vi "Action Worker Mode Example.vi"() -> ()   [LabVIEW 2017, in "Action Worker Mode Example.lvlib"]
uses:
  Action Worker Mode Example.lvlib
  user.lib/_NEVSTOP/Communicable State Machine(CSM)/_Support/Typedef/_CSM_Response Source Message.ctl
  user.lib/_NEVSTOP/Communicable State Machine(CSM)/_Support/Typedef/_CSM_MODE.ctl
  user.lib/_NEVSTOP/Communicable State Machine(CSM)/AdvanceAPI/CSM - Make String Arguments Safe.vi
  user.lib/_NEVSTOP/Communicable State Machine(CSM)/AdvanceAPI/CSM - Break Down Multiple States String.vi
  user.lib/_NEVSTOP/Communicable State Machine(CSM)/AdvanceAPI/CSM - Compact Multiple States.vi
  user.lib/_NEVSTOP/Communicable State Machine(CSM)/AdvanceAPI/CSM - Keywords.vi
  user.lib/_NEVSTOP/Communicable State Machine(CSM)/Communicable State Machine.lvlib
panel:
  in  "All?":bool
  out "Array":T2(array[cluster])
  out ">> Response Source Message >>":T3
  in  "DoSth: Error -> Worker":bool
  in  "DoSth: Error -@ Worker":bool
  in  "Macro: Exit -> Worker":bool
  in  "Macro: Exit -@ Worker":bool
  in  "DoSth: DoA -@ Worker":bool
  out "State History":string
  in  "DoSth: DoA -> Worker":bool
  # "Overview:\n\nThis demonstrates the worker mode in the CSM framework. Worker mode involves starting multiple clonable instances of CSM, which work together as sub-modules. Normally, if we use the same name for cloneable modules, a critical error will occur in the subsequently started instance. To distinguish it from normal cases, CSM uses a # postfix in module names. Suppose the workers are named with \"worker#\". If you try to send a message to \"worker\", the first idle instance will respond to the message. The term \"FIRST IDLE\" refers to using a fairy queue for waiting instances. From outside, you won't even know that 4 worker instances are running. All concepts of CSM remain unchanged in worker mode, including sync/async/status messages.\n\nIn this example, 4 worker instances of “worker” are running in the background. Please refer to the history log to identify which instance processed your message."
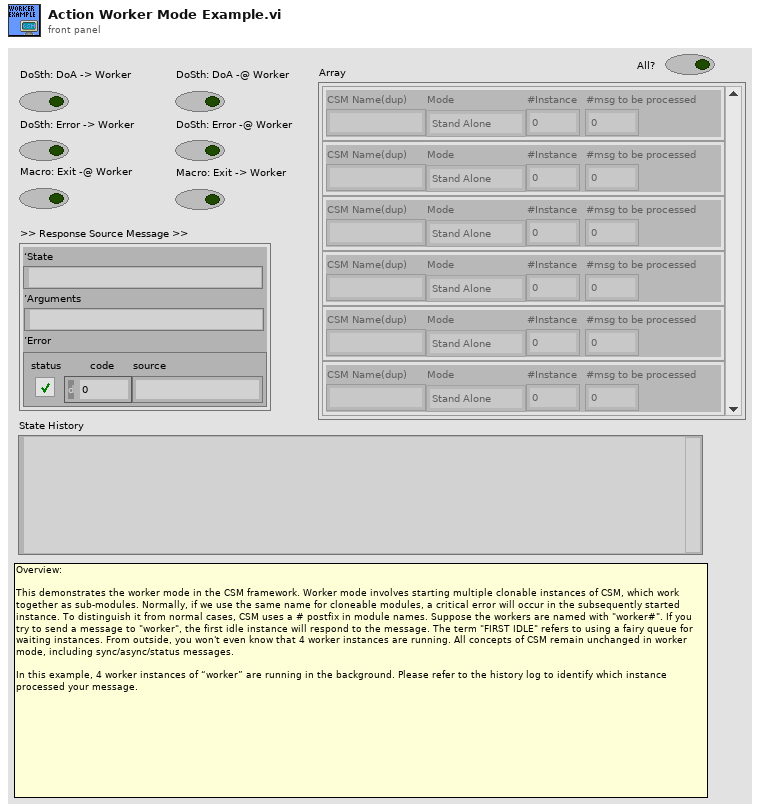
[diagram p1: front panel]
types:
  T1 = typedef "Communicable State Machine.lvlib/_CSM_MODE.ctl" = enum16{"Not Exist", "Stand Alone", "CSM", "Worker", "Worker Agent", "Chain Node", "Chain"}
  T2 = cluster{"CSM Name(dup)":string, "Mode":T1, "#Instance":i32, "#msg to be processed":i32}[]
  T3 = typedef "Communicable State Machine.lvlib/_CSM_Response Source Message.ctl" = cluster{"‘State":string, "’Arguments":string, "’Error":errorcluster}
  T4 = enum32{"Invalid", "Standard", "Closed", "Hidden", "Minimized", "Maximized"}
  T5 = enum32{"invalid app kind", "Development System", "Run Time System", "Student Edition", "Embedded LabVIEW", "Evaluation", "Custom"}
  T6 = cluster{"Current VI Reference":refnum<vi>, "Close Panel on Exit?":bool}
  T7 = cluster{"Core":cluster{"Current VI Reference":refnum<vi>, "Close Panel on Exit?":bool}, "Your Boolean data":bool, "Your string data":string}
  T8 = cluster{"CSM Name (Dup)":string, "Mode":T1, "#Instance":i32, "#Elements In Queue":i32}
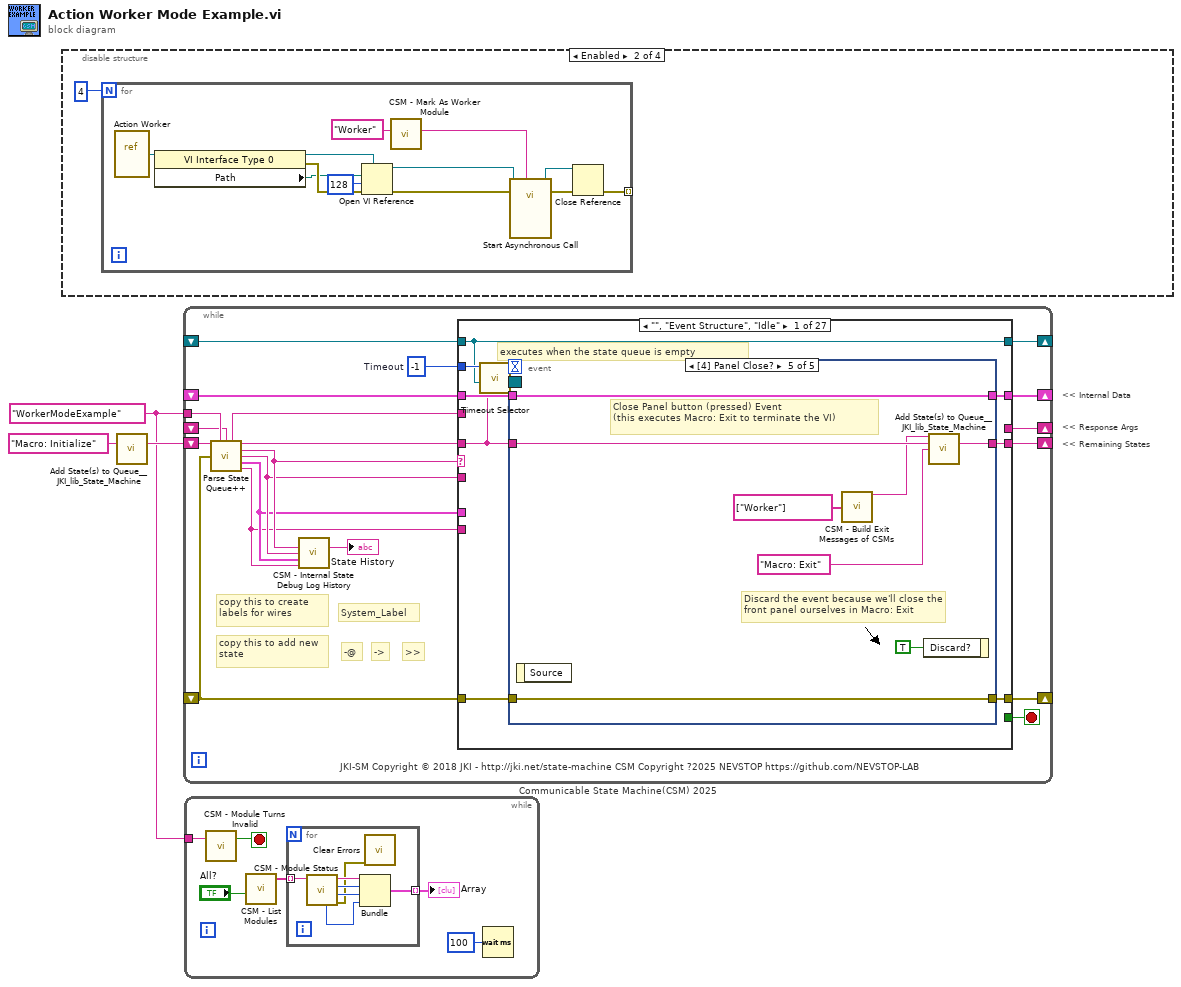
[diagram p0: block diagram]
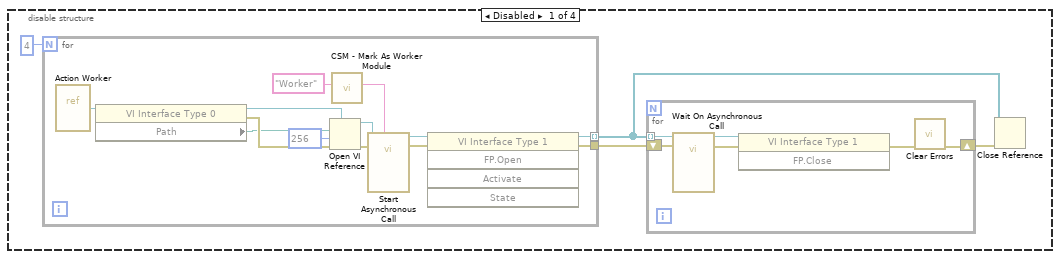
[diagram p2: hidden frame]
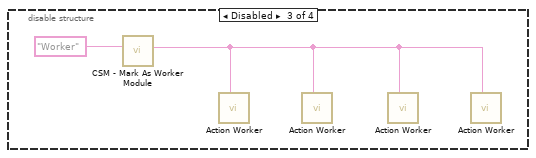
[diagram p3: hidden frame]
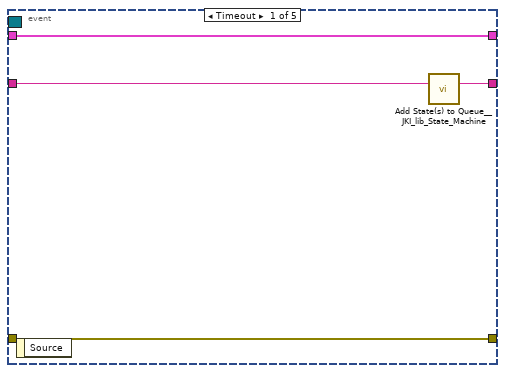
[diagram p5: hidden frame]
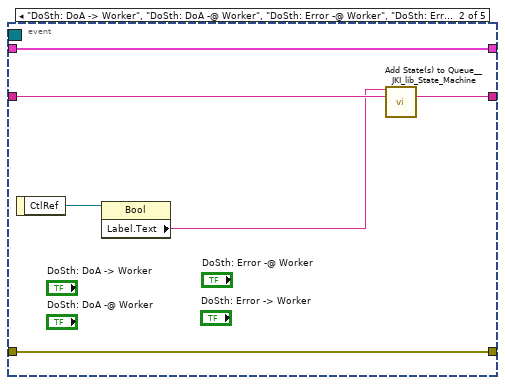
[diagram p6: hidden frame]
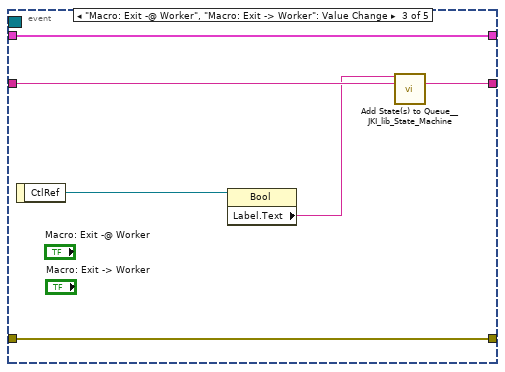
[diagram p7: hidden frame]
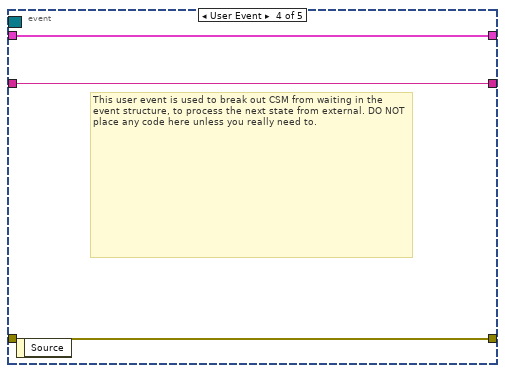
[diagram p8: hidden frame]
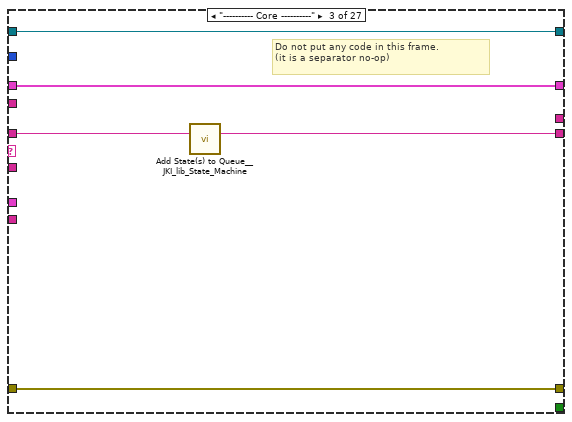
[diagram p10: hidden frame]
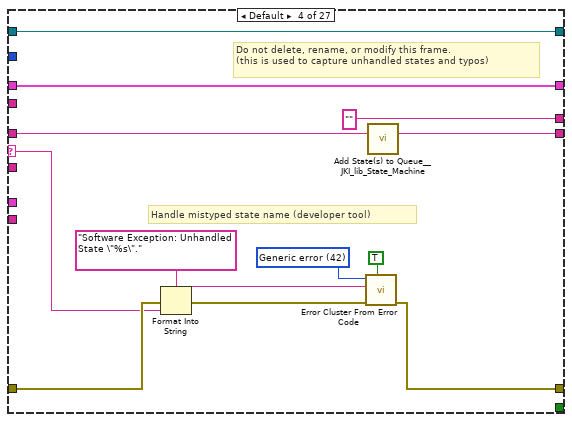
[diagram p11: hidden frame]
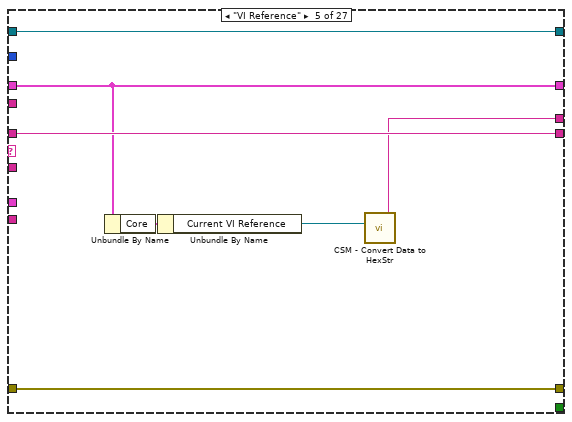
[diagram p12: hidden frame]
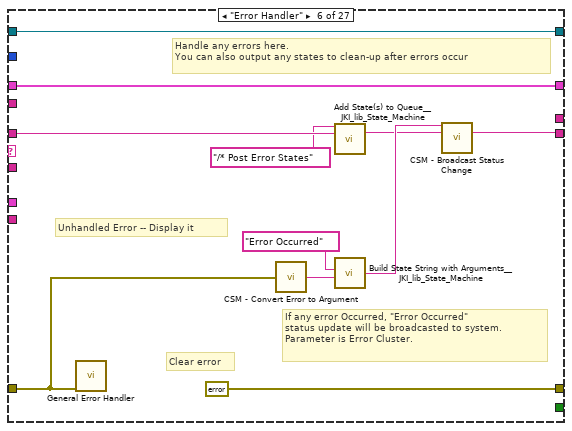
[diagram p13: hidden frame]
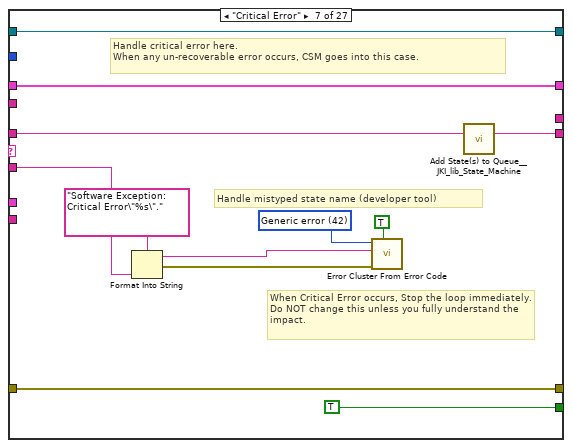
[diagram p14: hidden frame]
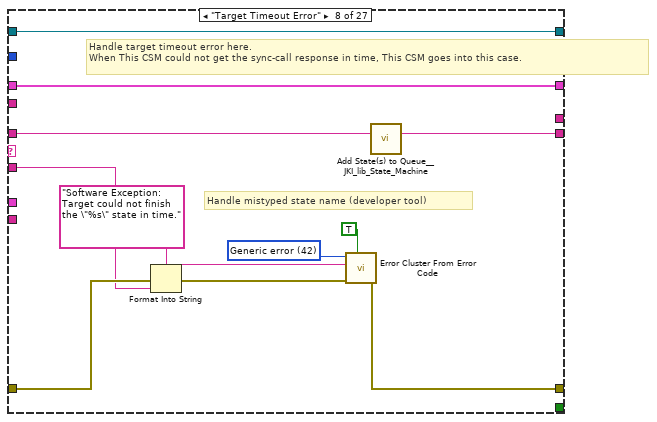
[diagram p15: hidden frame]
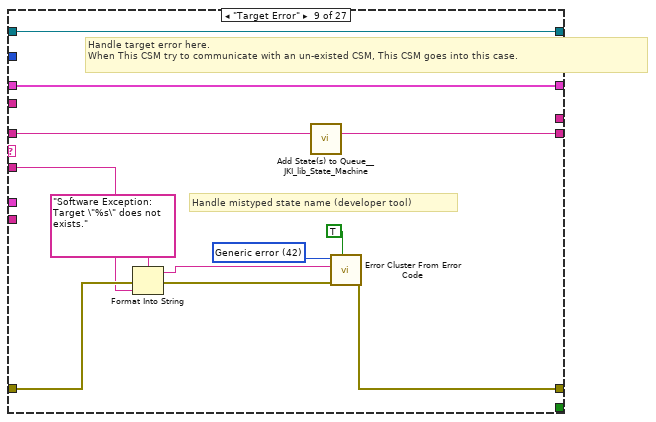
[diagram p16: hidden frame]
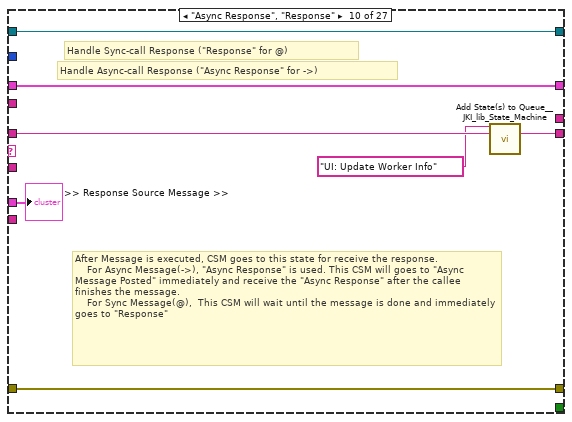
[diagram p17: hidden frame]
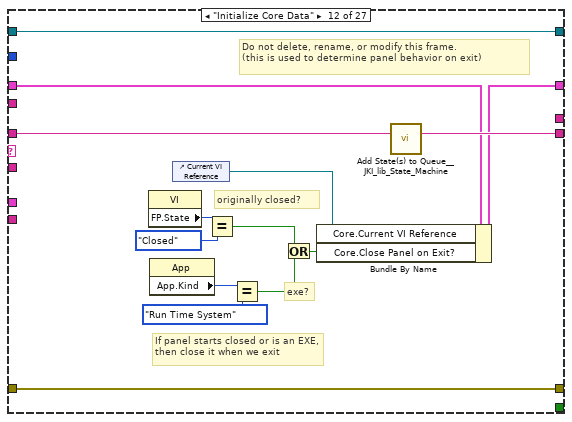
[diagram p19: hidden frame]
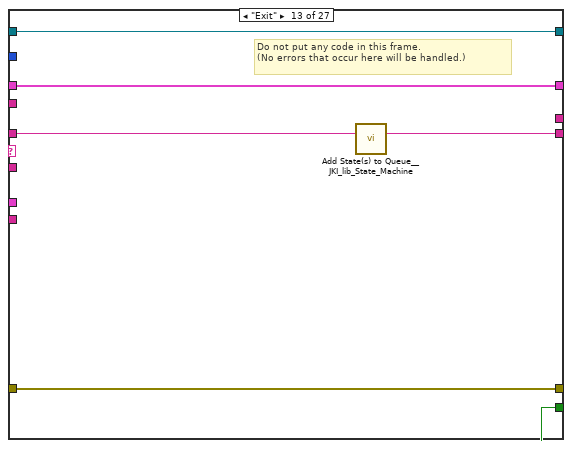
[diagram p20: hidden frame]
diagram:
  w1 = "WorkerModeExample" ("Name (\"\" to Use UUID)")
  # "<< Internal Data"
  # "<< Response Args"
  # "<< Remaining States"
  n1 = disable-structure shown="Enabled" {
    frame Disabled {
      n2 = for {
        N: 4 -> [_]
        tunnel: [w17] -> w4
        tunnel: [w18] -> w5 mode=indexing
        n3 = vi-ref "Action Worker.vi"() -> (w21:refnum<vi>)
        n4 = property class="VI Interface Type 0"(reference=w21) -> (reference out=w25:refnum<vi>, error out=w23:errorcluster, "Path"=w22:path)  [unwired: 1 in]
        n5 = Open VI Reference(type specifier VI Refnum (for type only)=w25, vi path=w22, options=256, error in (no error)=w23) -> (vi reference=w24:refnum<vi>, error out=w20:errorcluster)  [unwired: 2 in]
        n6 = call "CSM - Mark As Worker Module.vi"("CSM Name"="Worker" ("Name (\"\" to Use UUID)")) -> ("CSM Name (Marked As Worker)"=w14:string)  [unwired: 9 in]
        n7 = call-by-ref "Start Asynchronous Call"(reference=w24, error in=w20, "Name(\"\" to use uuid)"=w14) -> (reference out=w19:refnum<vi>, error out=w16:errorcluster)  [unwired: 11 in]
        n8 = invoke class="VI Interface Type 1" method="FP.Open"(reference=w19, error in=w16) -> (reference out=w18:refnum<vi>, error out=w17:errorcluster)  [unwired: 3 in, 3 out]
      }
      n9 = for {
        shift-right: [w8] -> w7
        shift-left: w4 -> [w13]
        tunnel: w5 -> [w12] mode=indexing
        n10 = call-by-ref "Wait On Asynchronous Call"(reference=w12, error in=w13) -> (reference out=w11:refnum<vi>, error out=w9:errorcluster)  [unwired: 12 in]
        n11 = invoke class="VI Interface Type 1" method="FP.Close"(reference=w11, error in=w9) -> (error out=w10:errorcluster)  [unwired: 1 in, 2 out]
        n12 = call <vilib>:"Clear Errors.vi"("error in (no error)"=w10) -> ("error out"=w8:errorcluster)  [unwired: 5 in, 1 out]
      }
      n13 = Close Reference(reference=w5, error in (no error)=w7) -> ()  [unwired: 1 out]
    }
    frame Enabled {
      n14 = for {
        N: 4 -> [_]
        tunnel: [w30] -> _ mode=indexing
        n15 = vi-ref "Action Worker.vi"() -> (w35:refnum<vi>)
        n16 = property class="VI Interface Type 0"(reference=w35) -> (reference out=w38:refnum<vi>, error out=w37:errorcluster, "Path"=w36:path)  [unwired: 1 in]
        n17 = Open VI Reference(type specifier VI Refnum (for type only)=w38, vi path=w36, options=128, error in (no error)=w37) -> (vi reference=w29:refnum<vi>, error out=w28:errorcluster)  [unwired: 2 in]
        n18 = call "CSM - Mark As Worker Module.vi"("CSM Name"="Worker" ("Name (\"\" to Use UUID)")) -> ("CSM Name (Marked As Worker)"=w33:string)  [unwired: 9 in]
        n19 = call-by-ref "Start Asynchronous Call"(reference=w29, error in=w28, "Name(\"\" to use uuid)"=w33) -> (reference out=w31:refnum<vi>, error out=w32:errorcluster)  [unwired: 11 in]
        n20 = Close Reference(reference=w31, error in (no error)=w32) -> (error out=w30:errorcluster)
      }
    }
    frame Disabled {
      n21 = call "CSM - Mark As Worker Module.vi"("CSM Name"="Worker" ("Name (\"\" to Use UUID)")) -> ("CSM Name (Marked As Worker)"=w40:string)  [unwired: 9 in]
      n22 = call "Action Worker.vi"("Name (\"\" to Use UUID)"=w40) -> ()  [unwired: 11 in]
      n23 = call "Action Worker.vi"("Name (\"\" to Use UUID)"=w40) -> ()  [unwired: 11 in]
      n24 = call "Action Worker.vi"("Name (\"\" to Use UUID)"=w40) -> ()  [unwired: 11 in]
      n25 = call "Action Worker.vi"("Name (\"\" to Use UUID)"=w40) -> ()  [unwired: 11 in]
    }
    frame Disabled {
    }
  }
  n26 = call <vilib>:"Add State(s) to Queue__JKI_lib_State_Machine.vi"("State(s) in (\"\")"="Macro: Initialize") -> ("States Out"=w3:string)  [unwired: 14 in]
  n27 = while "Communicable State Machine(CSM) 2025" {
    shift-right: [w56] -> _
    shift-left: _ -> [w55]
    shift-right: [w59] -> _
    shift-left: _ -> [w53]
    shift-right: [w58] -> _
    shift-left: w3 -> [w60]
    tunnel: w1 -> [w49]
    shift-right: [w52] -> _
    shift-left: _ -> [w43]
    shift-right: [w51] -> _
    shift-left: _ -> [w50]
    stop <- w57 stop-if-true
    w54 = -1  # Timeout
    # "JKI-SM Copyright © 2018 JKI - http://jki.net/state-machine CSM Copyright ?2025 NEVSTOP https://github.com/NEVSTOP-LAB"
    # "copy this to add new state"
    # ">>"
    # "->"
    # "-@"
    # "copy this to create labels for wires"
    # "System_Label"
    n28 = call "Parse State Queue++.vi"("State Queue"=w60, "Name (\"\" to Use UUID)"=w49, "Response Arguments"=w43, "Previous Error"=w53) -> ("Name Used"=w44:string, "Remaining States"=w61:string, "Current State"=w48:string, "Arguments"=w47:string, ">> Response Source Message >>"=w46:T3, ">> Source CSM >>"=w45:string)  [unwired: 6 in]
    n29 = call "CSM - Internal State Debug Log History.vi"("State"=w48, "Arguments (\"\")"=w47, ">> Response Source Message >>"=w46, "Source (\"\")"=w45) -> ("Debug Log"=→"State History":string)  [unwired: 11 in]
    n30 = case shown="\"\", \"Event Structure\", \"Idle\"" w48 {
      selector: w48 -> [_ _ _ w109 _ _ _ _ _ _ _ _ _ _ _ _ _ _ _ _ _ _ _ _ _ _ _]
      tunnel: w61 -> [w62 w100 w106 w113 w125 w137 w147 w155 w167 w177 w183 w198 w204 w209 w217 w224 w229 w235 w239 w245 w250 w257 w273 w341 w347 w353 w364]
      tunnel: w47 -> [_ _ _ _ _ _ w140 w151 w163 _ _ _ _ _ _ _ _ _ _ _ _ w252 w267 _ _ _ _]
      tunnel: w55 -> [w69 w99 w103 w111 w124 w135 w148 w153 w165 w179 w182 w191 w202 w206 _ w219 w226 w234 w238 w242 w248 w255 w269 w340 w344 w350 w361]
      tunnel: [w68 w101 w104 w115 w126 errorcluster {"status"=FALSE, "code"=0, "source"=""} ("error out") w149 w157 w169 w180 w184 w195 w201 w207 w214 w220 w227 w230 w237 w243 w247 w253 w270 w342 w345 w351 w362] -> w59
      tunnel: w53 -> [w67 w101 w104 w114 w126 w127 w149 w156 w168 w180 w184 w195 w201 w207 w214 w221 w227 _ w240 w243 w247 w254 w271 w342 w345 w351 w362]
      tunnel: [w70 w100 w105 w112 w125 w128 w146 w154 w166 w176 w183 w197 w203 w208 w216 w223 w228 w235 w239 w244 w249 w256 w272 w341 w346 w352 w363] -> w58
      tunnel: [_ _ _ _ _ _ TRUE _ _ _ _ _ TRUE _ _ _ _ _ _ _ _ _ _ _ _ _ _] -> w57
      tunnel: [w66 w99 w103 w111 w124 w135 w148 w153 w165 w179 w182 w196 w202 w206 w215 w219 w226 w234 w238 w242 w248 w255 w269 w340 w344 w350 w361] -> w56
      tunnel: w54 -> [w65 _ _ _ _ _ _ _ _ _ _ _ _ _ _ _ _ _ _ _ _ _ _ _ _ _ _]
      tunnel: w45 -> [_ _ _ _ _ _ _ _ _ _ _ _ _ _ _ _ _ _ _ _ _ _ _ _ _ _ _]
      tunnel: w46 -> [_ _ _ _ _ _ _ _ _ w174 _ _ _ _ _ _ _ _ _ _ _ _ _ _ _ _ _]
      tunnel: [_ _ _ "" w120 _ _ _ _ _ _ _ _ _ _ _ _ _ _ _ _ _ _ _ _ _ _] -> w52
      tunnel: [w64 w98 w102 w107 w123 w133 w138 w150 w162 w178 w181 w185 w199 w205 w210 w218 w225 w233 w236 w241 w246 w251 w266 w339 w343 w348 w354] -> w51
      tunnel: w50 -> [w64 w98 w102 w107 w123 w133 w138 w150 w162 w178 w181 w185 w199 w205 w210 w218 w225 _ w236 w241 w246 w251 w266 w339 w343 w348 w354]
      tunnel: w44 -> [_ _ _ _ _ _ _ _ _ _ _ _ _ _ _ _ _ w232 _ _ _ _ _ _ _ _ _]
      frame "", "Event Structure", "Idle" {
        # "executes when the state queue is empty"
        n31 = call "Timeout Selector.vi"("Remaining States"=w62, "Timeout Expected"=w65) -> ("Timeout"=w63:i32)  [unwired: 5 in]
        n32 = event shown="[4] Panel Close?" {
          selector: w64 -> [_ _ _ _ _]
          dyn-events: _ -> [_ _ _ _ _]
          timeout: w63 -> [_ _ _ _ _]
          tunnel: w62 -> [w74 w78 w84 w88 w97]
          tunnel: [w73 w77 w83 w88 w96] -> w70
          tunnel: w69 -> [w71 w79 w85 w89 w94]
          tunnel: [w72 w80 w86 w87 w95] -> w68
          tunnel: w67 -> [w72 w80 w86 w87 w95]
          tunnel: [w71 w79 w85 w89 w94] -> w66
          event Timeout {
            n33 = event-data() -> ()  [unwired: 1 in, 1 out]
            n34 = call <vilib>:"Add State(s) to Queue__JKI_lib_State_Machine.vi"("State(s) in (\"\")"=w74) -> ("States Out"=w73:string)  [unwired: 14 in]
          }
          event "DoSth: DoA -> Worker", "DoSth: DoA -@ Worker", "DoSth: Error -@ Worker", "DoSth: Error -> Worker": Value Change {
            n35 = event-data() -> ("CtlRef"=w76:refnum<vi>)  [unwired: 1 in]
            n36 = property class="Bool"(reference=w76) -> ("Label.Text"=w75:string)  [unwired: 1 in, 2 out]
            n37 = call <vilib>:"Add State(s) to Queue__JKI_lib_State_Machine.vi"("State(s) in Front (\"\")"=w75, "State(s) in (\"\")"=w78) -> ("States Out"=w77:string)  [unwired: 13 in]
          }
          event "Macro: Exit -@ Worker", "Macro: Exit -> Worker": Value Change {
            n38 = event-data() -> ("CtlRef"=w82:refnum<vi>)  [unwired: 1 in]
            n39 = property class="Bool"(reference=w82) -> ("Label.Text"=w81:string)  [unwired: 1 in, 2 out]
            n40 = call <vilib>:"Add State(s) to Queue__JKI_lib_State_Machine.vi"("State(s) in Front (\"\")"=w81, "State(s) in (\"\")"=w84) -> ("States Out"=w83:string)  [unwired: 13 in]
          }
          event User Event {
            # "This user event is used to break out CSM from waiting in the event structure, to process the next state from external. DO NOT place any code here unless you really need to."
            n41 = event-data() -> ()  [unwired: 1 in, 1 out]
          }
          event Panel Close? {
            # "Discard the event because we'll close the front panel ourselves in Macro: Exit"
            # "Close Panel button (pressed) Event\n(this executes Macro: Exit to terminate the VI)"
            n42 = event-data() -> ()  [unwired: 1 in, 1 out]
            n43 = call "CSM - Build Exit Messages of CSMs.vi"("CSMs"=string[] ["Worker"]) -> ("States"=w91:string)  [unwired: 14 in]
            n44 = event-data("Discard?"=TRUE) -> ()  [unwired: 1 in, 1 out]
            n45 = call <vilib>:"Add State(s) to Queue__JKI_lib_State_Machine.vi"("State(s) in Front (\"\")"=w91, "State(s) in (\"\")"=w97, "State(s) at Back (\"\")"="Macro: Exit") -> ("States Out"=w96:string)  [unwired: 12 in]
          }
        }
      }
      frame "CSM Documentation" {
        # "#CSM README FIRST\n\nCSM is a LabVIEW application framework that builds upon JKI State Machine (JKISM). It follows the pattern of JKISM and extends the keywords to describe message communication between CSM modules, including concepts such as Sync-Message, Async-Message, Subscription/Unsubscription of status - essential elements for creating reusable code modules. For more information, please visit the CSM wiki: https://github.com/NEVSTOP-LAB/JKI-State-Machine-Plus-Plus/wiki\n\nFor instructions on JKI State Machine, visit: http://jki.net/state-machine/\nFor information about CSM, visit: https://github.com/NEVSTOP-LAB"
        # "CSM Documentation"
      }
      frame "---------- Core ----------" {
        # "Do not put any code in this frame.\n(it is a separator no-op)"
        n46 = call <vilib>:"Add State(s) to Queue__JKI_lib_State_Machine.vi"("State(s) in (\"\")"=w106) -> ("States Out"=w105:string)  [unwired: 14 in]
      }
      frame Default {
        w118 = 42 items=["No error", "Argument error", "Memory is full", "Out of zone", "End of file", "File already open", "Generic file I/O error", "File not found", "File permission error", "Disk is full", "Duplicate path", "Too many files open", "System feature not enabled", "Resource file not found", "Cannot add resource", "Resource not found", "Image not found", "Image memory error", "Pen does not exist", "Config type invalid", "Config token not found", "Config parse error", "Config memory error", "Bad external code format", "Bad external code offset", "External code not present", "Null window", "Destroy window error", "Null menu", "Print aborted", "Bad print record", "Print driver error", "Windows error during printing", "Memory error during printing", "Print dialog error", "Generic print error", "Invalid device refnum", "Device not found", "Device parameter error", "Device unit error", "Cannot open device", "Device call aborted", "Generic error", "Cancelled by user", "Object ID too low", "Object ID too high", "Object not in heap", "Unknown heap", "Unknown object (invalid DefProc)", "Unknown object (DefProc not in table)", "Message out of range", "Invalid (null) method", "Unknown message", "Manager call not supported", "Bad address", "Network operation in progress", "Network operation timed out", "Connection is busy", "Network attribute not supported", "Network error", "Address in use", "System out of memory", "Connection aborted", "Connection refused", "Not connected", "Already connected", "Connection closed", "Initialization error (interapplication manager)", "Bad occurrence", "Wait on unbound occurrence handler", "Occurrence queue overflow", "Datalog type conflict", "Unused", "Unrecognized type (interapplication manager)", "Memory corrupt", "Failed to make temporary DLL", "Old CIN version", "Drag socket not found", "Failed to load drop-object", "Failed to register OLE object", "Failed to release OLE object", "Format specifier type mismatch", "Unknown format specifier", "Too few format specifiers", "Too many format specifiers", "Scan failed", "Newer CIN version", "Error converting to variant", "Runtime menu error", "Password tampered", "Variant attribute not found", "Incompatible variant data type", "Event data is not available", "Event Store is not present", "Occurrence is not found", "Event Queue is not created", "Event info is not available", "Refnum passed is NULL", "Error retrieving Class GUID", "Error retrieving CoClass GUID", "Error retrieving TypeLib GUID.", "Bad built application magic bytes.", "Specific driver is different from the specific driver associated with the Logical Name.", "There is no session opened to the class driver.", "Max Error", "MAX - Error with config objects", "MAX - Error loading configuration", "MAX - Group not supported"]
        # "Do not delete, rename, or modify this frame.\n(this is used to capture unhandled states and typos)"
        # "Handle mistyped state name (developer tool)"
        n47 = Format Into String(format string="Software Exception: Unhandled State \"%s\"." ("message"), error in=w114, w109) -> (resulting string=w117:string, error out=w116:errorcluster)  [unwired: 1 in]
        n48 = call <vilib>:"Error Cluster From Error Code.vi"("show call chain? (False)"=TRUE, "error in (no error)"=w116, "error message (\"\")"=w117, "error code (0)"=w118) -> ("error out"=w115:errorcluster)  [unwired: 5 in]
        n49 = call <vilib>:"Add State(s) to Queue__JKI_lib_State_Machine.vi"("State(s) in (\"\")"=w113) -> ("States Out"=w112:string)  [unwired: 14 in]
      }
      frame "VI Reference" {
        n50 = Unbundle By Name(w124) -> ("Core"=w122:T6)
        n51 = Unbundle By Name(w122) -> ("Current VI Reference"=w121:refnum<vi>)
        n52 = call "CSM - Convert Data to HexStr.vi"("Variant"=w121) -> ("HEX String (0-9,A-F)"=w120:string)  [unwired: 8 in]
      }
      frame "Error Handler" {
        # "If any error Occurred, \"Error Occurred\" \nstatus update will be broadcasted to system.\nParameter is Error Cluster."
        # "Unhandled Error -- Display it"
        # "Handle any errors here.\nYou can also output any states to clean-up after errors occur"
        # "Clear error"
        n53 = call <vilib>:"General Error Handler.vi"("error in (no error)"=w127) -> ()  [unwired: 10 in, 5 out]
        n54 = call "CSM - Convert Error to Argument.vi"("Error"=w127) -> ("Argument"=w131:string)  [unwired: 4 in]
        n55 = call <vilib>:"Add State(s) to Queue__JKI_lib_State_Machine.vi"("State(s) in Front (\"\")"="/* Post Error States", "State(s) in (\"\")"=w137) -> ("States Out"=w129:string)  [unwired: 13 in]
        n56 = call <vilib>:"Build State String with Arguments__JKI_lib_State_Machine.vi"("Arguments (\"\")"=w131, "State"="Error Occurred" ("Status with Arguments")) -> ("State with Arguments"=w130:string)  [unwired: 4 in]
        n57 = call "CSM - Broadcast Status Change.vi"("Status With Arguments"=w130, "State Queue"=w129) -> ("Remaining States"=w128:string)  [unwired: 13 in]
      }
      frame "Critical Error" {
        w144 = 42 items=["No error", "Argument error", "Memory is full", "Out of zone", "End of file", "File already open", "Generic file I/O error", "File not found", "File permission error", "Disk is full", "Duplicate path", "Too many files open", "System feature not enabled", "Resource file not found", "Cannot add resource", "Resource not found", "Image not found", "Image memory error", "Pen does not exist", "Config type invalid", "Config token not found", "Config parse error", "Config memory error", "Bad external code format", "Bad external code offset", "External code not present", "Null window", "Destroy window error", "Null menu", "Print aborted", "Bad print record", "Print driver error", "Windows error during printing", "Memory error during printing", "Print dialog error", "Generic print error", "Invalid device refnum", "Device not found", "Device parameter error", "Device unit error", "Cannot open device", "Device call aborted", "Generic error", "Cancelled by user", "Object ID too low", "Object ID too high", "Object not in heap", "Unknown heap", "Unknown object (invalid DefProc)", "Unknown object (DefProc not in table)", "Message out of range", "Invalid (null) method", "Unknown message", "Manager call not supported", "Bad address", "Network operation in progress", "Network operation timed out", "Connection is busy", "Network attribute not supported", "Network error", "Address in use", "System out of memory", "Connection aborted", "Connection refused", "Not connected", "Already connected", "Connection closed", "Initialization error (interapplication manager)", "Bad occurrence", "Wait on unbound occurrence handler", "Occurrence queue overflow", "Datalog type conflict", "Unused", "Unrecognized type (interapplication manager)", "Memory corrupt", "Failed to make temporary DLL", "Old CIN version", "Drag socket not found", "Failed to load drop-object", "Failed to register OLE object", "Failed to release OLE object", "Format specifier type mismatch", "Unknown format specifier", "Too few format specifiers", "Too many format specifiers", "Scan failed", "Newer CIN version", "Error converting to variant", "Runtime menu error", "Password tampered", "Variant attribute not found", "Incompatible variant data type", "Event data is not available", "Event Store is not present", "Occurrence is not found", "Event Queue is not created", "Event info is not available", "Refnum passed is NULL", "Error retrieving Class GUID", "Error retrieving CoClass GUID", "Error retrieving TypeLib GUID.", "Bad built application magic bytes.", "Specific driver is different from the specific driver associated with the Logical Name.", "There is no session opened to the class driver.", "Max Error", "MAX - Error with config objects", "MAX - Error loading configuration", "MAX - Group not supported"]
        # "Handle critical error here.\nWhen any un-recoverable error occurs, CSM goes into this case."
        # "When Critical Error occurs, Stop the loop immediately. Do NOT change this unless you fully understand the impact."
        # "Handle mistyped state name (developer tool)"
        n58 = Format Into String(format string="Software Exception: Critical Error\"%s\"." ("message"), w140) -> (resulting string=w143:string, error out=w142:errorcluster)  [unwired: 2 in]
        n59 = call <vilib>:"Error Cluster From Error Code.vi"("show call chain? (False)"=TRUE, "error in (no error)"=w142, "error message (\"\")"=w143, "error code (0)"=w144) -> ()  [unwired: 5 in, 1 out]
        n60 = call <vilib>:"Add State(s) to Queue__JKI_lib_State_Machine.vi"("State(s) in (\"\")"=w147) -> ("States Out"=w146:string)  [unwired: 14 in]
      }
      frame "Target Timeout Error" {
        w160 = 42 items=["No error", "Argument error", "Memory is full", "Out of zone", "End of file", "File already open", "Generic file I/O error", "File not found", "File permission error", "Disk is full", "Duplicate path", "Too many files open", "System feature not enabled", "Resource file not found", "Cannot add resource", "Resource not found", "Image not found", "Image memory error", "Pen does not exist", "Config type invalid", "Config token not found", "Config parse error", "Config memory error", "Bad external code format", "Bad external code offset", "External code not present", "Null window", "Destroy window error", "Null menu", "Print aborted", "Bad print record", "Print driver error", "Windows error during printing", "Memory error during printing", "Print dialog error", "Generic print error", "Invalid device refnum", "Device not found", "Device parameter error", "Device unit error", "Cannot open device", "Device call aborted", "Generic error", "Cancelled by user", "Object ID too low", "Object ID too high", "Object not in heap", "Unknown heap", "Unknown object (invalid DefProc)", "Unknown object (DefProc not in table)", "Message out of range", "Invalid (null) method", "Unknown message", "Manager call not supported", "Bad address", "Network operation in progress", "Network operation timed out", "Connection is busy", "Network attribute not supported", "Network error", "Address in use", "System out of memory", "Connection aborted", "Connection refused", "Not connected", "Already connected", "Connection closed", "Initialization error (interapplication manager)", "Bad occurrence", "Wait on unbound occurrence handler", "Occurrence queue overflow", "Datalog type conflict", "Unused", "Unrecognized type (interapplication manager)", "Memory corrupt", "Failed to make temporary DLL", "Old CIN version", "Drag socket not found", "Failed to load drop-object", "Failed to register OLE object", "Failed to release OLE object", "Format specifier type mismatch", "Unknown format specifier", "Too few format specifiers", "Too many format specifiers", "Scan failed", "Newer CIN version", "Error converting to variant", "Runtime menu error", "Password tampered", "Variant attribute not found", "Incompatible variant data type", "Event data is not available", "Event Store is not present", "Occurrence is not found", "Event Queue is not created", "Event info is not available", "Refnum passed is NULL", "Error retrieving Class GUID", "Error retrieving CoClass GUID", "Error retrieving TypeLib GUID.", "Bad built application magic bytes.", "Specific driver is different from the specific driver associated with the Logical Name.", "There is no session opened to the class driver.", "Max Error", "MAX - Error with config objects", "MAX - Error loading configuration", "MAX - Group not supported"]
        # "Handle target timeout error here.\nWhen This CSM could not get the sync-call response in time, This CSM goes into this case."
        # "Handle mistyped state name (developer tool)"
        n61 = Format Into String(format string="Software Exception: Target could not finish the \"%s\" state in time." ("message"), error in=w156, w151) -> (resulting string=w159:string, error out=w158:errorcluster)  [unwired: 1 in]
        n62 = call <vilib>:"Error Cluster From Error Code.vi"("show call chain? (False)"=TRUE, "error in (no error)"=w158, "error message (\"\")"=w159, "error code (0)"=w160) -> ("error out"=w157:errorcluster)  [unwired: 5 in]
        n63 = call <vilib>:"Add State(s) to Queue__JKI_lib_State_Machine.vi"("State(s) in (\"\")"=w155) -> ("States Out"=w154:string)  [unwired: 14 in]
      }
      frame "Target Error" {
        w172 = 42 items=["No error", "Argument error", "Memory is full", "Out of zone", "End of file", "File already open", "Generic file I/O error", "File not found", "File permission error", "Disk is full", "Duplicate path", "Too many files open", "System feature not enabled", "Resource file not found", "Cannot add resource", "Resource not found", "Image not found", "Image memory error", "Pen does not exist", "Config type invalid", "Config token not found", "Config parse error", "Config memory error", "Bad external code format", "Bad external code offset", "External code not present", "Null window", "Destroy window error", "Null menu", "Print aborted", "Bad print record", "Print driver error", "Windows error during printing", "Memory error during printing", "Print dialog error", "Generic print error", "Invalid device refnum", "Device not found", "Device parameter error", "Device unit error", "Cannot open device", "Device call aborted", "Generic error", "Cancelled by user", "Object ID too low", "Object ID too high", "Object not in heap", "Unknown heap", "Unknown object (invalid DefProc)", "Unknown object (DefProc not in table)", "Message out of range", "Invalid (null) method", "Unknown message", "Manager call not supported", "Bad address", "Network operation in progress", "Network operation timed out", "Connection is busy", "Network attribute not supported", "Network error", "Address in use", "System out of memory", "Connection aborted", "Connection refused", "Not connected", "Already connected", "Connection closed", "Initialization error (interapplication manager)", "Bad occurrence", "Wait on unbound occurrence handler", "Occurrence queue overflow", "Datalog type conflict", "Unused", "Unrecognized type (interapplication manager)", "Memory corrupt", "Failed to make temporary DLL", "Old CIN version", "Drag socket not found", "Failed to load drop-object", "Failed to register OLE object", "Failed to release OLE object", "Format specifier type mismatch", "Unknown format specifier", "Too few format specifiers", "Too many format specifiers", "Scan failed", "Newer CIN version", "Error converting to variant", "Runtime menu error", "Password tampered", "Variant attribute not found", "Incompatible variant data type", "Event data is not available", "Event Store is not present", "Occurrence is not found", "Event Queue is not created", "Event info is not available", "Refnum passed is NULL", "Error retrieving Class GUID", "Error retrieving CoClass GUID", "Error retrieving TypeLib GUID.", "Bad built application magic bytes.", "Specific driver is different from the specific driver associated with the Logical Name.", "There is no session opened to the class driver.", "Max Error", "MAX - Error with config objects", "MAX - Error loading configuration", "MAX - Group not supported"]
        # "Handle target error here.\nWhen This CSM try to communicate with an un-existed CSM, This CSM goes into this case."
        # "Handle mistyped state name (developer tool)"
        n64 = Format Into String(format string="Software Exception: Target \"%s\" does not exists." ("message"), error in=w168, w163) -> (resulting string=w171:string, error out=w170:errorcluster)  [unwired: 1 in]
        n65 = call <vilib>:"Add State(s) to Queue__JKI_lib_State_Machine.vi"("State(s) in (\"\")"=w167) -> ("States Out"=w166:string)  [unwired: 14 in]
        n66 = call <vilib>:"Error Cluster From Error Code.vi"("show call chain? (False)"=TRUE, "error in (no error)"=w170, "error message (\"\")"=w171, "error code (0)"=w172) -> ("error out"=w169:errorcluster)  [unwired: 5 in]
      }
      frame "Async Response", "Response" {
        # "Handle Async-call Response (\"Async Response\" for ->)"
        # "Handle Sync-call Response (\"Response\" for @)"
        # "After Message is executed, CSM goes to this state for receive the response. \n    For Async Message(->), \"Async Response\" is used. This CSM will goes to \"Async Message Posted\" immediately and receive the \"Async Response\" after the callee finishes the message.\n    For Sync Message(@),  This CSM will wait until the message is done and immediately goes to \"Response\""
        n67 = call <vilib>:"Add State(s) to Queue__JKI_lib_State_Machine.vi"("State(s) in Front (\"\")"="UI: Update Worker Info" ("State(s) at Back (\"\")"), "State(s) in (\"\")"=w177) -> ("States Out"=w176:string)  [unwired: 13 in]
        ">> Response Source Message >>" <- w174
      }
      frame "Async Message Posted" {
        # "Handle post action for async message (->)."
        # "After Async Message is posted (->), CSM goes to this state for post-action. You can use Argument - State to tell which Async Message is called."
      }
      frame "Initialize Core Data" {
        # "Do not delete, rename, or modify this frame.\n(this is used to determine panel behavior on exit)"
        # "originally closed?"
        # "exe?"
        # "If panel starts closed or is an EXE, then close it when we exit"
        n68 = property class="VI"() -> ("FP.State"=w188:T4)  [unwired: 2 in, 2 out]
        n69 = property class="App"() -> ("App.Kind"=w194:T5)  [unwired: 2 in, 2 out]
        n70 = control-ref of="Current VI Reference"() -> (w189:refnum<vi>)
        n71 = Equal?(x=w188, y=T4."Closed" ("Front Panel Window:State")) -> (x = y?=w186:bool)
        n72 = Equal?(x=w194, y=T5."Run Time System" ("Application:Kind")) -> (x = y?=w192:bool)
        n73 = Or(x=w186, y=w192) -> (x .or. y?=w190:bool)
        n74 = Bundle By Name(cluster=w191, "Core.Current VI Reference"=w189, "Core.Close Panel on Exit?"=w190) -> (w196:T7)
        n75 = call <vilib>:"Add State(s) to Queue__JKI_lib_State_Machine.vi"("State(s) in (\"\")"=w198) -> ("States Out"=w197:string)  [unwired: 14 in]
      }
      frame "Exit" {
        # "Do not put any code in this frame.\n(No errors that occur here will be handled.)"
        n76 = call <vilib>:"Add State(s) to Queue__JKI_lib_State_Machine.vi"("State(s) in (\"\")"=w204) -> ("States Out"=w203:string)  [unwired: 14 in]
      }
      frame "---------- Data ----------" {
        # "Do not put any code in this frame.\n(It is a separator no-op. You can make a copy of this frame to create a new Data frame)"
        n77 = call <vilib>:"Add State(s) to Queue__JKI_lib_State_Machine.vi"("State(s) in (\"\")"=w209) -> ("States Out"=w208:string)  [unwired: 14 in]
      }
      frame "Data: Initialize" {
        w211 = T6 {"Current VI Reference"=refnum, "Close Panel on Exit?"=FALSE}  # Core
        w213 = TRUE  # Your Boolean data
        w212 = ""  # Your string data
        # "do not delete - used by framework"
        # "Expand Bundle to add new data elements to shift register data."
        # "Add new data here."
        # "Initialize the shift-register data, here.\n(data names are defined by what you wire into the bundle function)"
        n78 = Bundle("Core"=w211, "Your Boolean data"=w213, "Your string data"=w212) -> (w215:T7)  [unwired: 1 in]
        n79 = call <vilib>:"Add State(s) to Queue__JKI_lib_State_Machine.vi"("State(s) in (\"\")"=w217) -> ("States Out"=w216:string)  [unwired: 14 in]
      }
      frame "Data: Cleanup" {
        # "Cleanup any data and references, here.\n(this is called automatically, by the Macro: Exit)"
        n80 = Unbundle By Name(w219) -> ("Core.Current VI Reference"=w222:refnum<vi>)
        n81 = Close Reference(reference=w222, error in (no error)=w221) -> (error out=w220:errorcluster)
        n82 = call <vilib>:"Add State(s) to Queue__JKI_lib_State_Machine.vi"("State(s) in (\"\")"=w224) -> ("States Out"=w223:string)  [unwired: 14 in]
      }
      frame "---------- Events ----------" {
        # "Do not put any code in this frame.\n(It is a separator no-op. You can make a copy of this frame to create a new UI frame)"
        n83 = call <vilib>:"Add State(s) to Queue__JKI_lib_State_Machine.vi"("State(s) in (\"\")"=w229) -> ("States Out"=w228:string)  [unwired: 14 in]
      }
      frame "Events: Register" {
        # "Register message event to break Waiting in Event structure."
        n84 = call "CSM - Get New State Notifier Event.vi"("Name (\"\" to Use UUID) In"=w232) -> ("error out"=w230:errorcluster, "New State Notifier Event"=w231:refnum<user-event>)  [unwired: 9 in]
        n85 = register-events(w231) -> (reference out=w233:refnum<event-registration>)  [unwired: 2 in, 1 out]
      }
      frame "Events: Unregister" {
        n86 = Unregister For Events(event registration refnum=w236, error in=w240) -> (error out=w237:errorcluster)
      }
      frame "---------- UI ----------" {
        # "Do not put any code in this frame.\n(It is a separator no-op. You can make a copy of this frame to create a new UI frame)"
        n87 = call <vilib>:"Add State(s) to Queue__JKI_lib_State_Machine.vi"("State(s) in (\"\")"=w245) -> ("States Out"=w244:string)  [unwired: 14 in]
      }
      frame "UI: Initialize" {
        # "Initialize the User Interface, here.\n(this is called automatically, by the Macro: Init)"
        n88 = call <vilib>:"Add State(s) to Queue__JKI_lib_State_Machine.vi"("State(s) in (\"\")"=w250) -> ("States Out"=w249:string)  [unwired: 14 in]
      }
      frame "UI: Cursor Set" {
        # "Argument"
        # "Set and Unset Cursor Busy.\n(Usage: \"UI: Cursor Set >> Busy|Idle\")"
        n89 = disable-structure shown="Default" {
          disable-tunnel: w254 -> [w260 w265]
          disable-tunnel: [w259 w265] -> w253
          disable-tunnel: w252 -> [w258 _]
          frame condition #0 (active) {
            n90 = case shown="\"Idle\", Default" w258 {
              tunnel: w260 -> [w262 w264]
              tunnel: [w261 w263] -> w259
              frame "Idle", Default {
                n91 = call <vilib>:"Unset Busy.vi"("error in (no error)"=w262) -> ("error out"=w261:errorcluster)  [unwired: 10 in]
              }
              frame "Busy" {
                n92 = call <vilib>:"Set Busy.vi"("error in (no error)"=w264) -> ("error out"=w263:errorcluster)  [unwired: 9 in, 1 out]
              }
            }
          }
          frame condition #1 {
          }
        }
        n93 = call <vilib>:"Add State(s) to Queue__JKI_lib_State_Machine.vi"("State(s) in (\"\")"=w257) -> ("States Out"=w256:string)  [unwired: 14 in]
      }
      frame "UI: Front Panel State" {
        # "Argument"
        # "Set Front Panel Open or Closed\n(Usage: \"UI: Front Panel State >> Open|Close\")"
        n94 = Unbundle By Name(w269) -> ("Core.Current VI Reference"=w268:refnum<vi>)
        n95 = call <vilib>:"Add State(s) to Queue__JKI_lib_State_Machine.vi"("State(s) in (\"\")"=w273) -> ("States Out"=w272:string)  [unwired: 14 in]
        n96 = case shown="\"Minimize\", \"Minimized\"" w267 {
          tunnel: w271 -> [w279 w294 w305 w318 w331]
          tunnel: [w281 w295 w307 w320 w333] -> w270
          tunnel: w268 -> [w280 w292 w306 w319 w332]
          frame "Open", "Standard", Default {
            w274 = T4."Standard" ("State")
            n97 = property class="VI"(reference=w280, error in=w279) -> (reference out=w277:refnum<vi>, error out=w278:errorcluster, "FP.State"=w276:T4)
            n98 = Not Equal?(x=w276, y=w274) -> (x != y?=w275:bool)
            n99 = case shown="True" w275 {
              tunnel: [w285 w287] -> w281
              tunnel: w278 -> [w284 w287]
              tunnel: w277 -> [w283 _]
              tunnel: w274 -> [w282 _]
              frame True {
                n100 = invoke class="VI" method="FP.Open"(reference=w283, error in=w284, "Activate"=TRUE, "State"=w282) -> (error out=w285:errorcluster)  [unwired: 1 in, 4 out]
              }
              frame False {
              }
            }
          }
          frame "Close", "Closed" {
            n101 = property class="VI"(reference=w292, error in=w294) -> (reference out=w291:refnum<vi>, error out=w293:errorcluster, "FP.State"=w289:T4)
            n102 = Not Equal?(x=w289, y=T4."Closed" ("Front Panel Window:State")) -> (x != y?=w288:bool)
            n103 = case shown="True" w288 {
              tunnel: [w296 w299] -> w295
              tunnel: w293 -> [w296 w298]
              tunnel: w291 -> [_ w297]
              frame False {
              }
              frame True {
                n104 = invoke class="VI" method="FP.Close"(reference=w297, error in=w298) -> (error out=w299:errorcluster)  [unwired: 1 in, 2 out]
              }
            }
          }
          frame "Hidden", "Hide" {
            w300 = T4."Hidden" ("State")
            n105 = property class="VI"(reference=w306, error in=w305) -> (reference out=w303:refnum<vi>, error out=w304:errorcluster, "FP.State"=w302:T4)
            n106 = Not Equal?(x=w302, y=w300) -> (x != y?=w301:bool)
            n107 = case shown="True" w301 {
              tunnel: [w311 w312] -> w307
              tunnel: w304 -> [w310 w312]
              tunnel: w303 -> [w309 _]
              tunnel: w300 -> [w308 _]
              frame True {
                n108 = invoke class="VI" method="FP.Open"(reference=w309, error in=w310, "State"=w308) -> (error out=w311:errorcluster)  [unwired: 2 in, 4 out]
              }
              frame False {
              }
            }
          }
          frame "Minimize", "Minimized" {
            w313 = T4."Minimized" ("State")
            n109 = property class="VI"(reference=w319, error in=w318) -> (reference out=w316:refnum<vi>, error out=w317:errorcluster, "FP.State"=w315:T4)
            n110 = Not Equal?(x=w315, y=w313) -> (x != y?=w314:bool)
            n111 = case shown="True" w314 {
              tunnel: [w324 w325] -> w320
              tunnel: w317 -> [w323 w325]
              tunnel: w316 -> [w322 _]
              tunnel: w313 -> [w321 _]
              frame True {
                n112 = invoke class="VI" method="FP.Open"(reference=w322, error in=w323, "State"=w321) -> (error out=w324:errorcluster)  [unwired: 2 in, 4 out]
              }
              frame False {
              }
            }
          }
          frame "Maximize", "Maximized" {
            w326 = T4."Maximized" ("State")
            n113 = property class="VI"(reference=w332, error in=w331) -> (reference out=w329:refnum<vi>, error out=w330:errorcluster, "FP.State"=w328:T4)
            n114 = Not Equal?(x=w328, y=w326) -> (x != y?=w327:bool)
            n115 = case shown="True" w327 {
              tunnel: [w337 w338] -> w333
              tunnel: w330 -> [w336 w338]
              tunnel: w329 -> [w335 _]
              tunnel: w326 -> [w334 _]
              frame True {
                n116 = invoke class="VI" method="FP.Open"(reference=w335, error in=w336, "State"=w334) -> (error out=w337:errorcluster)  [unwired: 2 in, 4 out]
              }
              frame False {
              }
            }
          }
        }
      }
      frame "UI: Update Worker Info" {
      }
      frame "---------- Macro ----------" {
        # "Do not put any code in this frame.\n(It is a separator no-op. You can make a copy of this frame to create a new Macro frame)"
        n117 = call <vilib>:"Add State(s) to Queue__JKI_lib_State_Machine.vi"("State(s) in (\"\")"=w347) -> ("States Out"=w346:string)  [unwired: 14 in]
      }
      frame "Macro: Initialize" {
        w349 = "Data: Initialize\nInitialize Core Data\nEvents: Register\nUI: Initialize\nUI: Front Panel State >> Open\nUI: Update Worker Info"  # Data: Initialize Initialize Core Data Events: Register UI: Initialize UI: Front Panel State >> Open UI: Update Worker Info
        # "Initialization Macro\n(This is called once, when the VI starts)"
        n118 = call <vilib>:"Add State(s) to Queue__JKI_lib_State_Machine.vi"("State(s) in Front (\"\")"=w349, "State(s) in (\"\")"=w353) -> ("States Out"=w352:string)  [unwired: 13 in]
      }
      frame "Macro: Exit" {
        # "Exit Macro\n(This is called once, when the VI exits)"
        n119 = Unbundle By Name(w361) -> ("Core.Close Panel on Exit?"=w360:bool)
        n120 = Select(t="UI: Front Panel State >> Close", s=w360, f="") -> (s? t:f=w357:string)
        n121 = call <vilib>:"Add State(s) to Queue__JKI_lib_State_Machine.vi"("State(s) in (\"\")"=w357, "State(s) at Back (\"\")"="Data: Cleanup\nEvents: Unregister\nExit") -> ("States Out"=w355:string)  [unwired: 13 in]
        n122 = call <vilib>:"Add State(s) to Queue__JKI_lib_State_Machine.vi"("State(s) in Front (\"\")"=w355, "State(s) in (\"\")"=w364) -> ("States Out"=w363:string)  [unwired: 13 in]
      }
    }
  }
  n123 = while {
    tunnel: w1 -> [w367]
    stop <- w368 stop-if-true
    n124 = call "CSM - Module Turns Invalid.vi"("CSM Name"=w367) -> ("Turn Invalid (Exit)?"=w368:bool)  [unwired: 2 in]
    n125 = call "CSM - List Modules.vi"("With Instance? (F)"="All?") -> ("Module Names"=w369:string[])  [unwired: 9 in, 1 out]
    n126 = for {
      tunnel: w369 -> [w377] mode=indexing
      tunnel: [w372] -> w370 mode=indexing
      n127 = call "CSM - Module Status.vi"("CSM Name"=w377) -> ("error out"=w371:errorcluster, "#Instance"=w374:i32, "Mode"=w375:T1, "CSM Name (Dup)"=w376:string, "#Elements In Queue"=w373:i32)  [unwired: 6 in]
      n128 = Bundle("CSM Name (Dup)"=w376, "Mode"=w375, "#Instance"=w374, "#Elements In Queue"=w373) -> (w372:T8)  [unwired: 1 in]
      n129 = call <vilib>:"Clear Errors.vi"("error in (no error)"=w371) -> ()  [unwired: 5 in, 2 out]
    }
    "Array" <- w370
    n130 = Wait (ms)(milliseconds to wait=u32 100) -> ()  [unwired: 1 out]
  }
